vi "DIO_CH0_CH4.vi"() -> ()   [LabVIEW 2018]
panel:
  out "AI1":dbl(graph)
  out "AI0":dbl[](graph)
  in  "DIO4":bool
  out "DIO0":bool
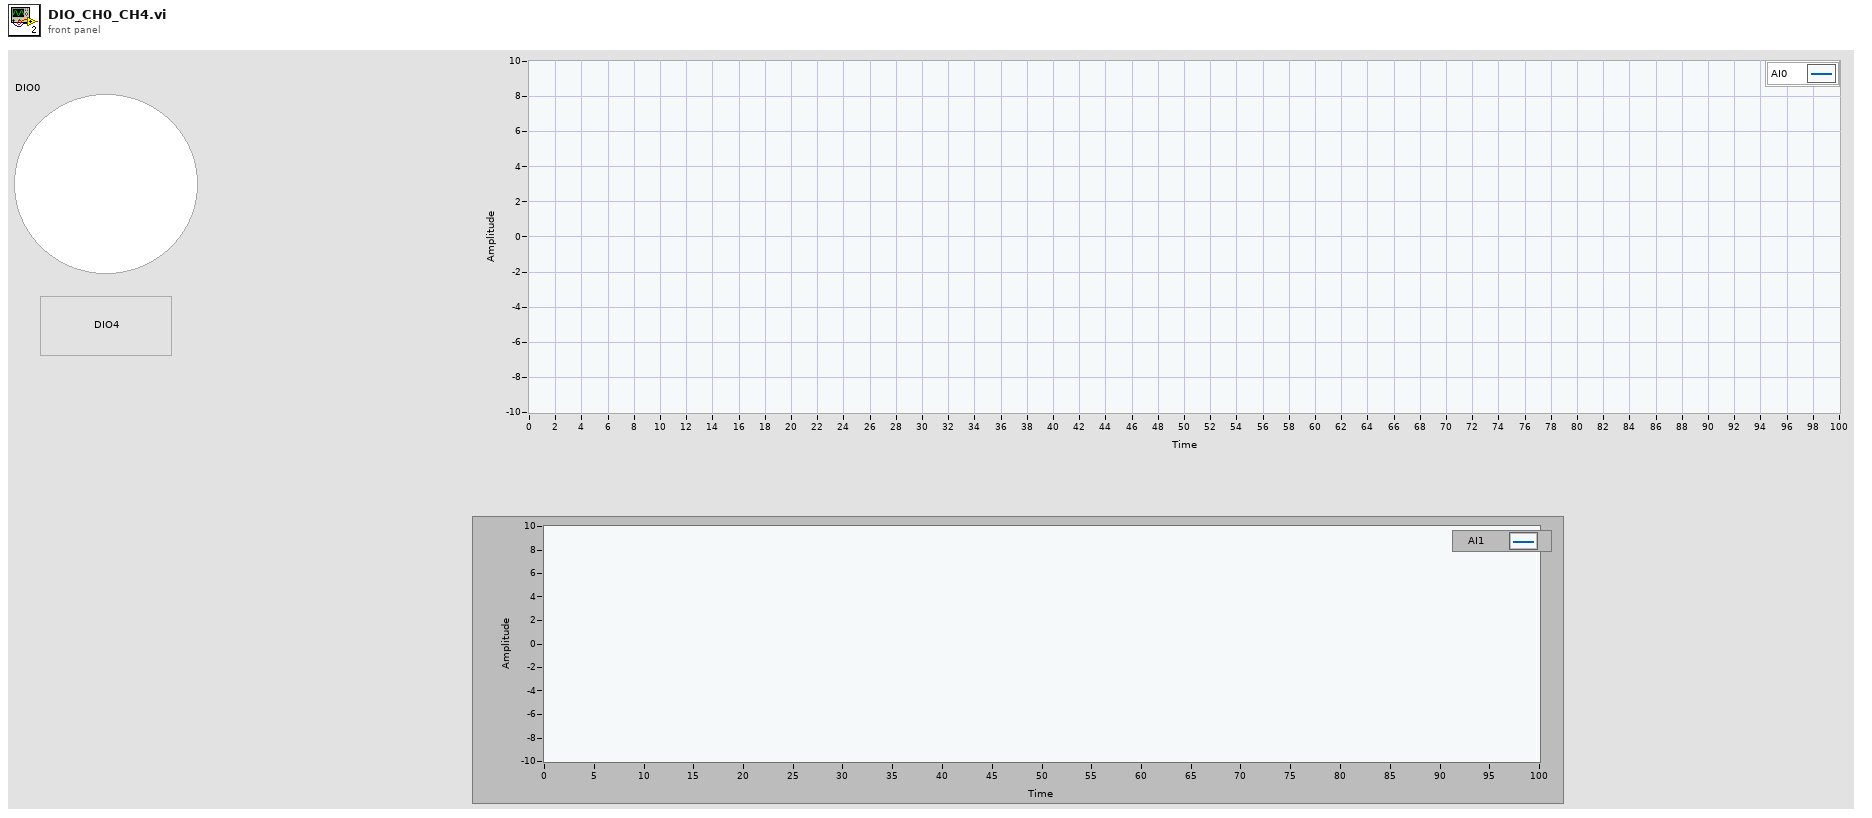
[diagram p1: front panel]
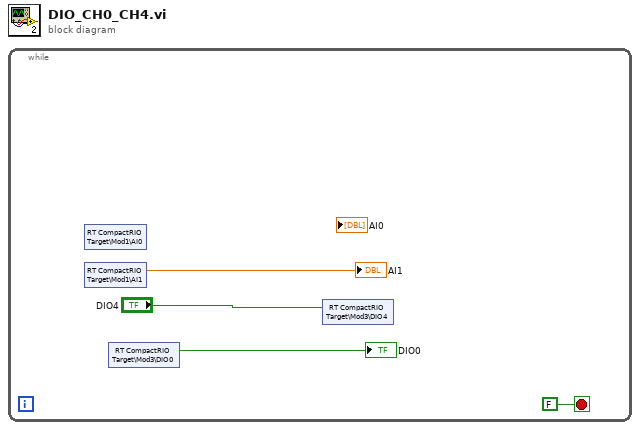
[diagram p0: block diagram]
diagram:
  n1 = while {
    stop <- FALSE stop-if-true
    n2 = shared-variable "RT CompactRIO Target\\Mod1\\AI0"() -> ()  [unwired: 1 in, 2 out]
    n3 = shared-variable "RT CompactRIO Target\\Mod1\\AI1"() -> (→"AI1":dbl)  [unwired: 1 in, 1 out]
    n4 = shared-variable "RT CompactRIO Target\\Mod3\\DIO0"() -> (→"DIO0":bool)  [unwired: 1 in, 1 out]
    n5 = shared-variable "RT CompactRIO Target\\Mod3\\DIO4"("DIO4") -> ()  [unwired: 1 in, 1 out]
  }
